vi "jMsg_TCPClient_Connection_Update (create).vi"(8 "error in (no error)":errorcluster, 10 "IP Address":string, 11 "Port":u16) -> (0 "error out":errorcluster, 3 "jMsg_TCPClient_Connection_Update":refnum<class "jMsg_TCPClient_Connection_Update.lvclass">)   [LabVIEW 2019, in "jMsg_TCPClient_Connection_Update.lvclass"]
doc: "This VI is used to create the jMsg\n\n\nJSMA Message Wizard 0.2.0.5\nRob Humfeld - Jet Engineering\nCopyright (c) 2020, Jet Engineering"
uses:
  jMsg_TCPClient_Connection_Update.lvclass
  C:/Program Files/National Instruments/LabVIEW 2019/user.lib/Jet Engineering/JSMA/Libraries/jMsg Class/jMsg.lvclass
  <userlib>/Jet Engineering/JSMA/Libraries/jMsg Class/jMsg.lvclass/jMsg.ctl
  jMsg_TCPClient_Connection_Update.lvclass/jMsg_TCPClient_Connection_Update.ctl
  <userlib>/Jet Engineering/JSMA/Libraries/Shared/JSMA_GetClassName.vi
  <vilib>/Utility/LVClass/Get LV Class Path.vi
  <userlib>/Jet Engineering/JSMA/Libraries/jMsg Class/jMsg.lvclass
panel:
  in  "jMsg_TCPClient_Connection_Update":refnum<class "jMsg_TCPClient_Connection_Update.lvclass">
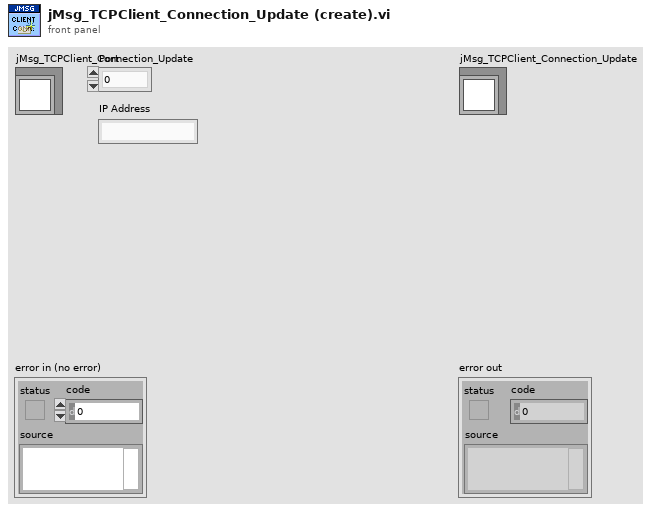
[diagram p1: front panel]
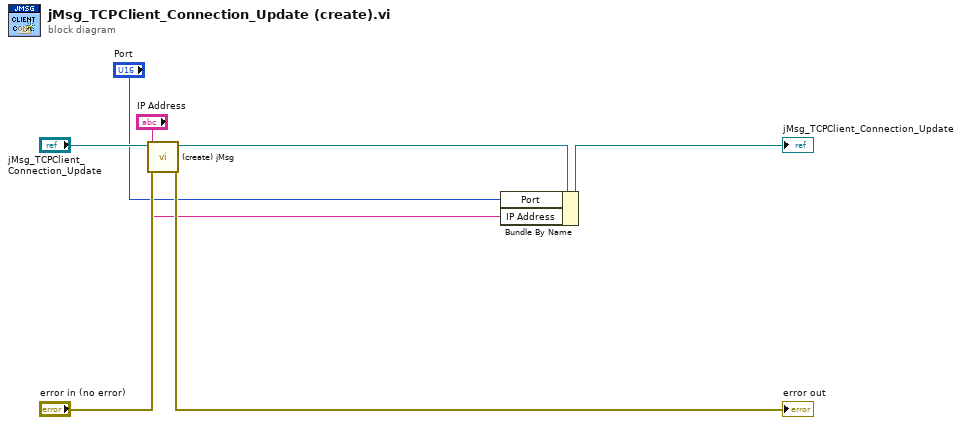
[diagram p0: block diagram]
diagram:
  n1 = call <userlib>:"(create) jMsg.vi"("error in (no error)"="error in (no error)", "jMsg in"="jMsg_TCPClient_Connection_Update") -> ("error out"=→"error out":errorcluster, "jMsg out"=w3:refnum<class "jMsg_TCPClient_Connection_Update.lvclass">)  [unwired: 8 in]
  n2 = Bundle By Name(cluster=w3, "Port"="Port", "IP Address"="IP Address") -> (→"jMsg_TCPClient_Connection_Update":refnum<class "jMsg_TCPClient_Connection_Update.lvclass">)
